vi "AxesControl.vi"(0 "Axis Up Down":string, 1 "Axis Left Right":string, 2 "Step size":dbl, 3 "Axis Up Down 2":string, 4 "Step size 2":dbl) -> ()   [LabVIEW 2014]
doc: "This VI allows the user to perform relative motion with a user defined step size of all every connected axis.\nThe VI sends messages in the name \"PI_Main\" queue that is also used by the FastAlignment_GUI as the main application.\nThis VI was designed for reentrant execution to allow the user to control more than three axes at once."
uses:
  C:/ProgramData/PI/LabVIEW/Low Level/General command.llb/Controller names.ctl
  Message Cluster.ctl
  C:/ProgramData/PI/LabVIEW/Low Level/General command.llb/Global2 (Array).vi
panel:
  out "Controller name":T1
  in  "stop":bool
  in  "System no.":i32=1 min=1 step=1
  in  "Up Down 2 Axis":u16(ring) items=["1", "2", "3", "4", "5", "6", "7", "8", "9", "10", "11", "12"]
  in  "Up Down Axis":u16(ring) items=["1", "2", "3", "4", "5", "6", "7", "8", "9", "10", "11", "12"]
  in  "Left Right Axis":u16(ring) items=["1", "2", "3", "4", "5", "6", "7", "8", "9", "10", "11", "12"]
  in  "Down Button 2":bool
  in  "Up Button 2":bool
  in  "Up Button":bool
  in  "Right Button":bool
  in  "Left Button":bool
  in  "Down Button":bool
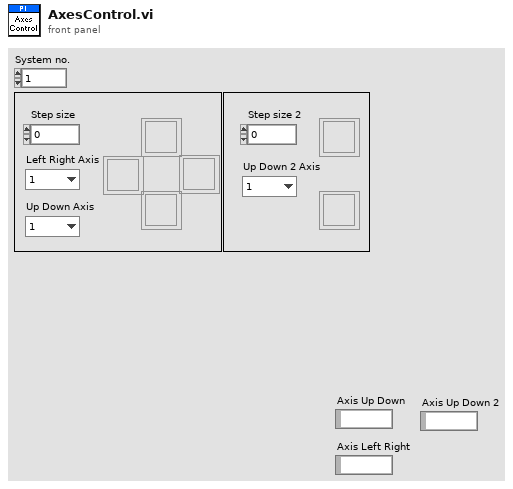
[diagram p1: front panel]
types:
  T1 = typedef "Controller names.ctl" = enum16{"None", "Analog", "C-702", "C-413", "C-414", "C-843", "C-843.PM", "C-844", "C-848", "C-865", "C-866", "C-867", "C-877", "C-880", "C-884", "C-885", "C-886", "C-887", "C-891", "E-135", "E-516", "E-517", "E-518", "E-709", "E-710", "E-712", "E-725", "E-727", "E-753", "E-754", "E-755", "E-761", "E-816", "E-861", "E-870", "E-871", "E-872", "E-873", "E-874", "F-206", "HydraPollux", "M-840", "M-850", "M-8X0", "Mercury", "Mercury_GCS", "PI_GCS2"}
  T2 = typedef "Message Cluster.ctl" = cluster{"Message":string, "Message Data":variant}
  T3 = cluster{"Conn. axes":string[], "Controller name":T1}[]
  T4 = cluster{"Conn. axes":string[], "Controller name":T1}
  T5 = cluster{"Axis":string, "Target":dbl, "System no.":i32}
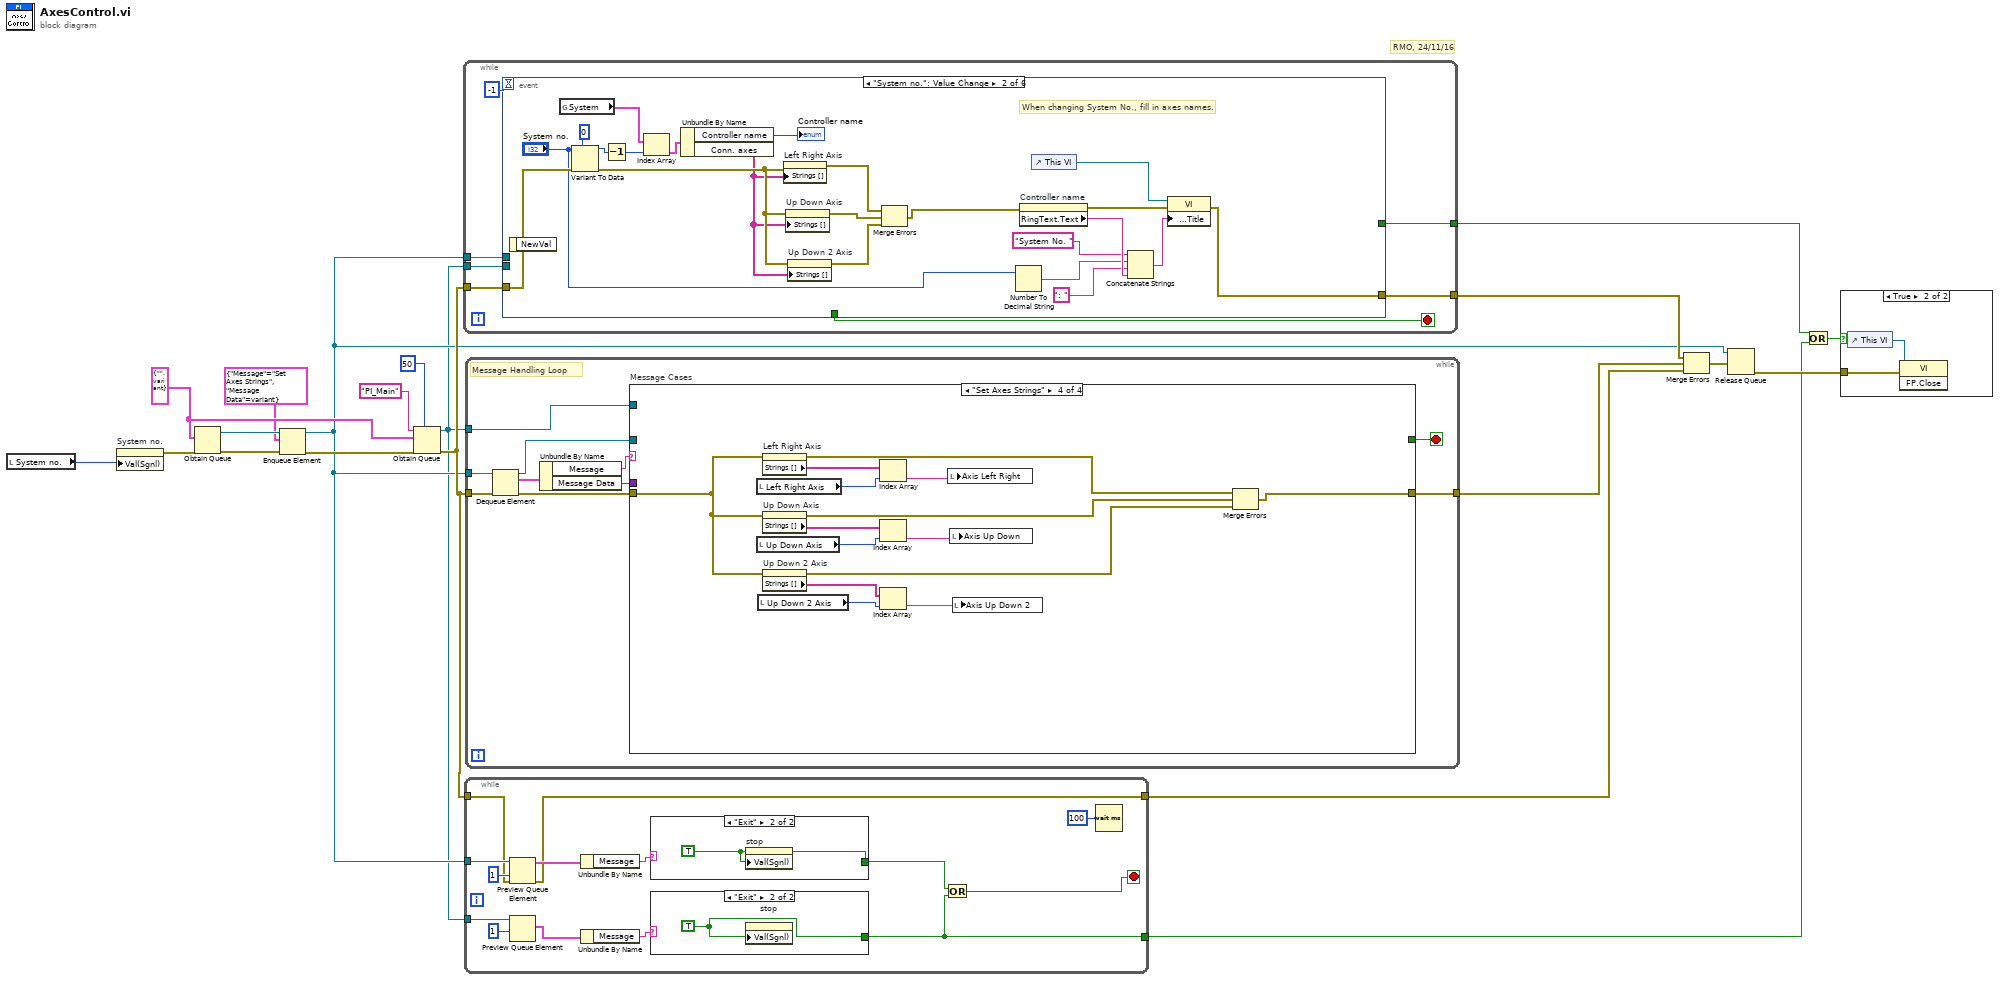
[diagram p0: block diagram]
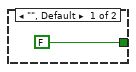
[diagram p3: hidden frame]
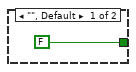
[diagram p4: hidden frame]
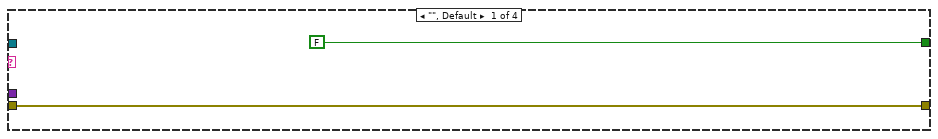
[diagram p5: hidden frame]
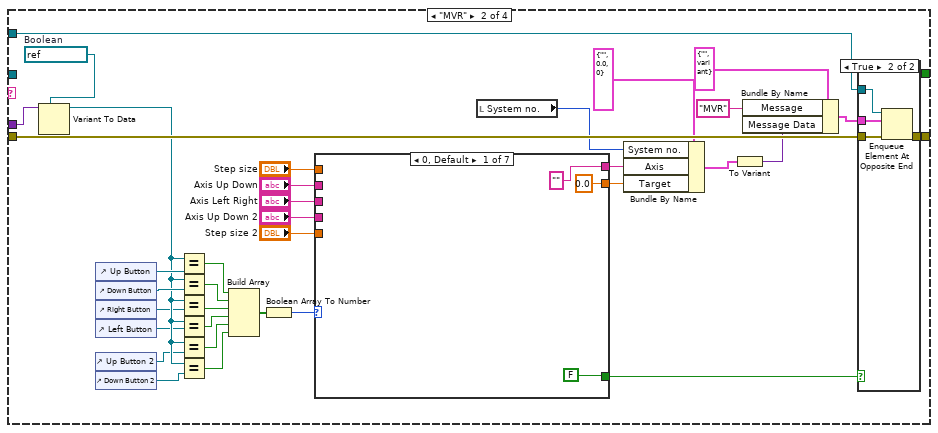
[diagram p6: hidden frame]
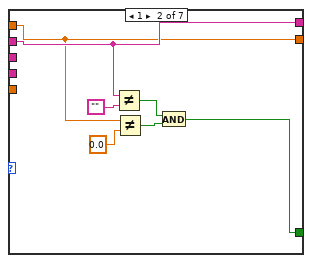
[diagram p8: hidden frame]
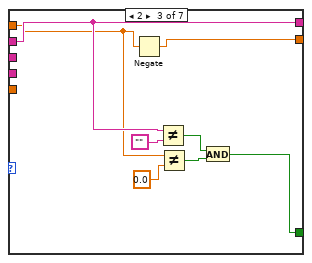
[diagram p9: hidden frame]
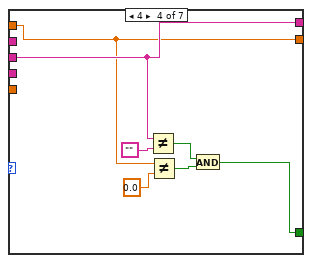
[diagram p10: hidden frame]
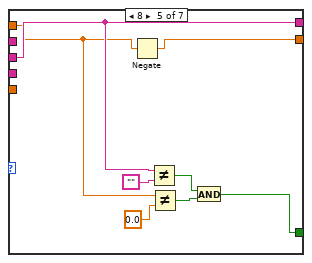
[diagram p11: hidden frame]
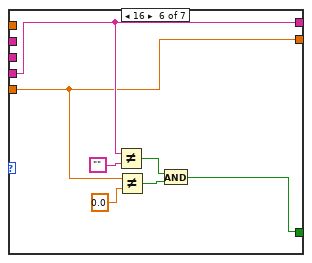
[diagram p12: hidden frame]
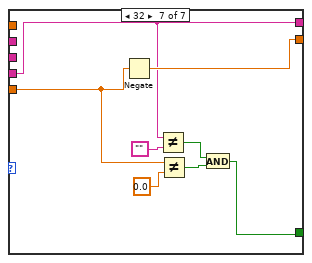
[diagram p13: hidden frame]
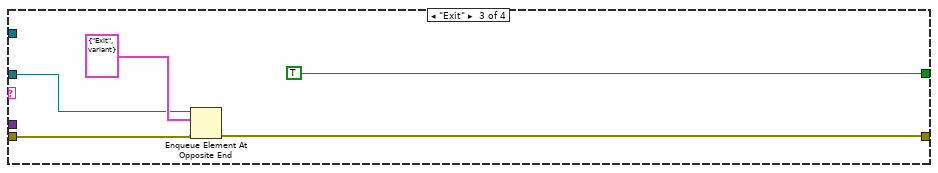
[diagram p14: hidden frame]
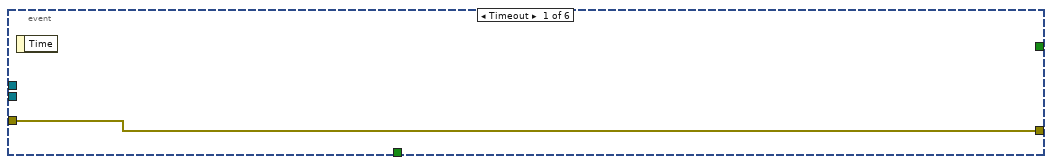
[diagram p15: hidden frame]
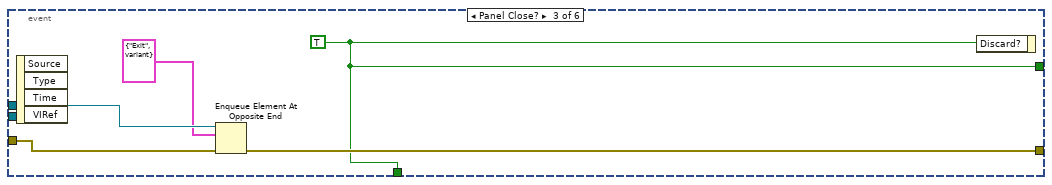
[diagram p16: hidden frame]
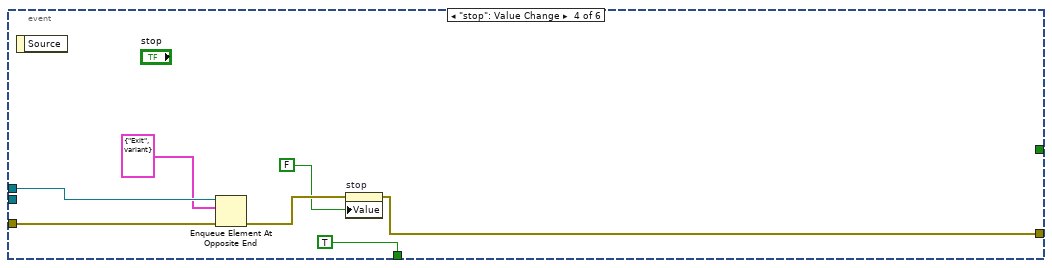
[diagram p17: hidden frame]
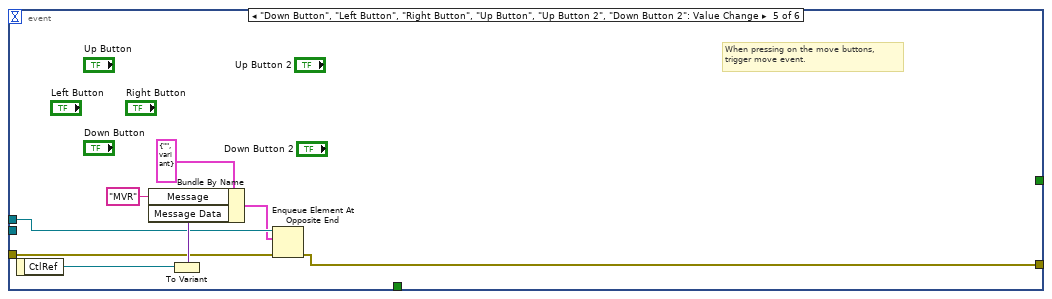
[diagram p18: hidden frame]
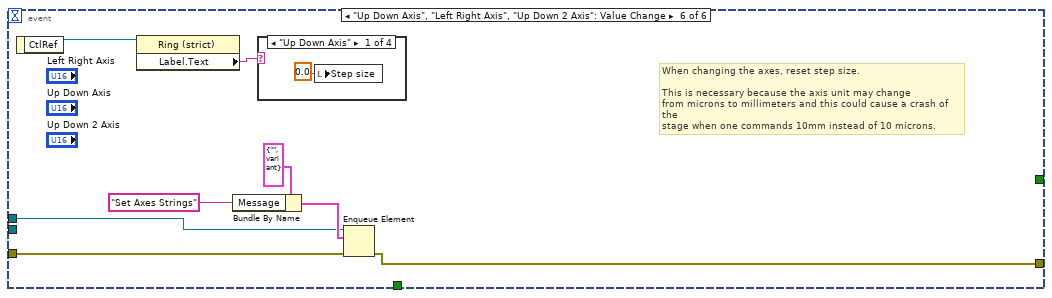
[diagram p19: hidden frame]
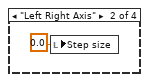
[diagram p20: hidden frame]
diagram:
  w18 = T2 {"Message"="", "Message Data"=variant} ("Message Cluster")
  # "RMO, 24/11/16"
  n1 = local read "System no."() -> (w1:i32)
  n2 = property on="System no." class="DigNum (strict)"("Val(Sgnl)"=w1) -> (error out=w2:errorcluster)  [unwired: 2 in, 1 out]
  n3 = Obtain Queue(element data type=w18, error in (no error)=w2) -> (queue out=w14:refnum<queue>, error out=w15:errorcluster)  [unwired: 2 in, 2 out]
  n4 = Enqueue Element(queue=w14, element=T2 {"Message"="Set Axes Strings", "Message Data"=variant} ("Message Cluster"), error in (no error)=w15) -> (queue out=w7:refnum<queue>, error out=w13:errorcluster)  [unwired: 2 out]
  n5 = Obtain Queue(max queue size (-1, unlimited)=50, name (unnamed)="PI_Main", element data type=w18, error in (no error)=w13) -> (queue out=w6:refnum<queue>, error out=w9:errorcluster)  [unwired: 1 in, 1 out]
  n6 = while {
    tunnel: [w27] -> w19
    tunnel: w6 -> [w26]
    tunnel: w9 -> [w24]
    tunnel: w7 -> [w22]
    tunnel: [w21] -> w5
    stop <- w25 stop-if-true
    n7 = event shown="[1] \"System no.\": Value Change" {
      selector: _ -> [_ _ _ _ _ _]
      dyn-events: _ -> [_ _ _ _ _ _]
      timeout: -1 -> [_ _ _ _ _ _]
      tunnel: [w28 w31 w53 w57 w70 w76] -> w27
      tunnel: w26 -> [_ _ _ _ _ _]
      tunnel: [_ _ w51 TRUE _ _] -> w25
      tunnel: w24 -> [w28 w40 w54 w61 w63 w74]
      tunnel: w22 -> [_ _ w55 w62 w66 w75]
      tunnel: [_ _ w51 _ _ _] -> w21
      event Timeout {
        n8 = event-data() -> ()  [unwired: 2 out]
      }
      event "System no.": Value Change {
        # "When changing System No., fill in axes names."
        n9 = event-data() -> ()  [unwired: 2 out]
        n10 = global read "Global2 (Array).vi" "System"() -> (w42:T3)
        n11 = Variant To Data(error in=w40, type=0, Variant="System no.") -> (data=w44:i32, error out=w47:errorcluster)
        n12 = Decrement(x=w44) -> (x-1=w45:i32)
        n13 = Index Array(array=w42, index=w45) -> (element=w43:T4)
        n14 = Unbundle By Name(w43) -> ("Controller name"=→"Controller name":T1, "Conn. axes"=w46:string[])
        n15 = property on="Left Right Axis" class="Ring (strict)"(error in=w47, "Strings []"=w46) -> (error out=w48:errorcluster)  [unwired: 1 in, 1 out]
        n16 = property on="Up Down Axis" class="Ring (strict)"(error in=w47, "Strings []"=w46) -> (error out=w49:errorcluster)  [unwired: 1 in, 1 out]
        n17 = property on="Up Down 2 Axis" class="Ring (strict)"(error in=w47, "Strings []"=w46) -> (error out=w50:errorcluster)  [unwired: 1 in, 1 out]
        n18 = Merge Errors(w48, w49, w50) -> (w32:errorcluster)
        n19 = Number To Decimal String(number="System no.") -> (decimal integer string=w36:string)  [unwired: 1 out]
        n20 = property on="Controller name" class="Enum (strict)"(error in=w32) -> (error out=w34:errorcluster, "RingText.Text"=w39:string)  [unwired: 1 in, 1 out]
        n21 = control-ref of="This VI"() -> (w33:refnum<vi>)
        n22 = Concatenate Strings("System No. ", w36, ": " ("string"), w39) -> (w38:string)
        n23 = property class="VI"(reference=w33, error in=w34, "Front Panel.Title"=w38) -> (error out=w31:errorcluster)  [unwired: 1 out]
      }
      event Panel Close? {
        w51 = TRUE
        n24 = event-data() -> ()  [unwired: 5 out]
        n25 = Enqueue Element At Opposite End(queue=w55, element=T2 {"Message"="Exit", "Message Data"=variant}, error in (no error)=w54) -> (error out=w53:errorcluster)  [unwired: 3 out]
        n26 = event-data("Discard?"=w51) -> ()  [unwired: 1 in, 1 out]
      }
      event "stop": Value Change {
        n27 = event-data() -> ()  [unwired: 2 out]
        n28 = Enqueue Element At Opposite End(queue=w62, element=T2 {"Message"="Exit", "Message Data"=variant}, error in (no error)=w61) -> (error out=w59:errorcluster)  [unwired: 3 out]
        n29 = property on="stop" class="Bool (strict)"(error in=w59, "Value"=FALSE) -> (error out=w57:errorcluster)  [unwired: 1 in, 1 out]
      }
      event "Down Button", "Left Button", "Right Button", "Up Button", "Up Button 2", "Down Button 2": Value Change {
        # "When pressing on the move buttons,\ntrigger move event."
        n30 = event-data() -> ("CtlRef"=w64:refnum<vi>)  [unwired: 1 out]
        n31 = To Variant(anything=w64) -> (Variant=w68:variant)
        n32 = Bundle By Name(cluster=T2 {"Message"="", "Message Data"=variant} ("Message Cluster"), "Message"="MVR", "Message Data"=w68) -> (w65:T2)
        n33 = Enqueue Element At Opposite End(queue=w66, element=w65, error in (no error)=w63) -> (error out=w70:errorcluster)  [unwired: 3 out]
      }
      event "Up Down Axis", "Left Right Axis", "Up Down 2 Axis": Value Change {
        # "When changing the axes, reset step size.\n\nThis is necessary because the axis unit may change\nfrom microns to millimeters and this could cause a crash of the\nstage when one commands 10mm instead of 10 microns."
        n34 = event-data() -> ("CtlRef"=w72:refnum<vi>)  [unwired: 1 out]
        n35 = property class="Ring (strict)"(reference=w72) -> ("Label.Text"=w71:string)  [unwired: 1 in, 2 out]
        n36 = Bundle By Name(cluster=T2 {"Message"="", "Message Data"=variant} ("Message Cluster"), "Message"="Set Axes Strings") -> (w77:T2)
        n37 = case shown="\"Up Down Axis\"" w71 {
          frame "Up Down Axis" {
            n38 = local write "Step size"(0.0 ("Step size")) -> ()
          }
          frame "Left Right Axis" {
            n39 = local write "Step size"(0.0 ("Step size")) -> ()
          }
          frame "", Default {
          }
          frame "Up Down 2 Axis" {
            n40 = local write "Step size 2"(0.0 ("Step size")) -> ()
          }
        }
        n41 = Enqueue Element(queue=w75, element=w77, error in (no error)=w74) -> (error out=w76:errorcluster)  [unwired: 3 out]
      }
    }
  }
  n42 = while {
    tunnel: w7 -> [w92]
    tunnel: w9 -> [w90]
    tunnel: [w89] -> w8
    tunnel: w6 -> [w85]
    tunnel: [w82] -> w4
    stop <- w86 stop-if-true
    n43 = Preview Queue Element(queue=w92, timeout in ms (-1)=1, error in (no error)=w90) -> (element=w95:T2, error out=w89:errorcluster)  [unwired: 2 out]
    n44 = Preview Queue Element(queue=w85, timeout in ms (-1)=1) -> (element=w84:T2)  [unwired: 1 in, 3 out]
    n45 = Unbundle By Name(w95) -> ("Message"=w94:string)
    n46 = Unbundle By Name(w84) -> ("Message"=w88:string)
    n47 = case shown="\"Exit\"" w94 {
      tunnel: [FALSE w99] -> w87
      frame "", Default {
      }
      frame "Exit" {
        w99 = TRUE
        n48 = property on="stop" class="Bool (strict)"("Val(Sgnl)"=w99) -> ()  [unwired: 2 in, 2 out]
      }
    }
    n49 = case shown="\"Exit\"" w88 {
      tunnel: [FALSE w97] -> w82
      frame "", Default {
      }
      frame "Exit" {
        w97 = TRUE
        n50 = property on="stop" class="Bool (strict)"("Val(Sgnl)"=w97) -> ()  [unwired: 2 in, 2 out]
      }
    }
    n51 = Or(x=w87, y=w82) -> (x .or. y?=w86:bool)
    n52 = Wait (ms)(milliseconds to wait=u32 100) -> ()  [unwired: 1 out]
  }
  n53 = while {
    tunnel: w7 -> [w101]
    tunnel: w9 -> [w107]
    tunnel: [w108] -> w17
    tunnel: w6 -> [w102]
    stop <- w109 stop-if-true
    # "Message Handling Loop"
    n54 = Dequeue Element(queue=w101, error in (no error)=w107) -> (queue out=w100:refnum<queue>, element=w106:T2, error out=w105:errorcluster)  [unwired: 2 out]
    n55 = Unbundle By Name(w106) -> ("Message"=w104:string, "Message Data"=w103:variant)
    n56 = case "Message Cases" shown="\"Set Axes Strings\"" w104 {
      tunnel: w105 -> [w111 w146 w203 w212]
      tunnel: [w111 w145 w202 w205] -> w108
      tunnel: [FALSE _ TRUE _] -> w109
      tunnel: w103 -> [_ w135 _ _]
      tunnel: w102 -> [_ w144 _ _]
      tunnel: w100 -> [_ _ w200 _]
      frame "", Default {
      }
      frame "MVR" {
        w137 = refnum<vi> refnum  # Boolean
        n57 = Variant To Data(type=w137, Variant=w135) -> (data=w133:refnum<vi>)  [unwired: 1 in, 1 out]
        n58 = control-ref of="Up Button"() -> (w136:refnum<vi>)
        n59 = control-ref of="Down Button"() -> (w134:refnum<vi>)
        n60 = control-ref of="Right Button"() -> (w114:refnum<vi>)
        n61 = control-ref of="Left Button"() -> (w113:refnum<vi>)
        n62 = control-ref of="Up Button 2"() -> (w118:refnum<vi>)
        n63 = control-ref of="Down Button 2"() -> (w117:refnum<vi>)
        n64 = Equal?(x=w133, y=w136) -> (x = y?=w132:bool)
        n65 = Equal?(x=w133, y=w134) -> (x = y?=w131:bool)
        n66 = Equal?(x=w133, y=w114) -> (x = y?=w130:bool)
        n67 = Equal?(x=w133, y=w113) -> (x = y?=w129:bool)
        n68 = Equal?(x=w133, y=w118) -> (x = y?=w128:bool)
        n69 = Equal?(x=w133, y=w117) -> (x = y?=w127:bool)
        n70 = Build Array(w132, w131, w130, w129, w128, w127) -> (w126:bool[])
        n71 = Boolean Array To Number(Boolean array=w126) -> (number=w122:u32)
        n72 = case shown="0, Default" w122 {
          tunnel: "Step size" -> [_ w156 w163 w171 w178 _ _]
          tunnel: "Axis Up Down" -> [_ w157 w164 _ _ _ _]
          tunnel: "Axis Left Right" -> [_ _ _ w172 w179 _ _]
          tunnel: "Axis Up Down 2" -> [_ _ _ _ _ w187 w194]
          tunnel: "Step size 2" -> [_ _ _ _ _ w186 w193]
          tunnel: [FALSE w155 w162 w170 w177 w185 w192] -> w121
          tunnel: ["" w157 w164 w172 w179 w187 w194] -> w116
          tunnel: [0.0 ("Step size 2") w156 w169 w171 w184 w186 w199] -> w115
          frame 0, Default {
          }
          frame 1 {
            n73 = Not Equal?(x=w157, y="") -> (x != y?=w159:bool)
            n74 = Not Equal?(x=w156, y=0.0 ("Step size")) -> (x != y?=w158:bool)
            n75 = And(x=w159, y=w158) -> (x .and. y?=w155:bool)
          }
          frame 2 {
            n76 = Negate(x=w163) -> (-x=w169:dbl)
            n77 = Not Equal?(x=w164, y="") -> (x != y?=w166:bool)
            n78 = Not Equal?(x=w163, y=0.0 ("Step size")) -> (x != y?=w165:bool)
            n79 = And(x=w166, y=w165) -> (x .and. y?=w162:bool)
          }
          frame 4 {
            n80 = Not Equal?(x=w172, y="") -> (x != y?=w174:bool)
            n81 = Not Equal?(x=w171, y=0.0 ("Step size")) -> (x != y?=w173:bool)
            n82 = And(x=w174, y=w173) -> (x .and. y?=w170:bool)
          }
          frame 8 {
            n83 = Negate(x=w178) -> (-x=w184:dbl)
            n84 = Not Equal?(x=w179, y="") -> (x != y?=w181:bool)
            n85 = Not Equal?(x=w178, y=0.0 ("Step size")) -> (x != y?=w180:bool)
            n86 = And(x=w181, y=w180) -> (x .and. y?=w177:bool)
          }
          frame 16 {
            n87 = Not Equal?(x=w187, y="") -> (x != y?=w189:bool)
            n88 = Not Equal?(x=w186, y=0.0 ("Step size")) -> (x != y?=w188:bool)
            n89 = And(x=w189, y=w188) -> (x .and. y?=w185:bool)
          }
          frame 32 {
            n90 = Negate(x=w193) -> (-x=w199:dbl)
            n91 = Not Equal?(x=w194, y="") -> (x != y?=w196:bool)
            n92 = Not Equal?(x=w193, y=0.0 ("Step size")) -> (x != y?=w195:bool)
            n93 = And(x=w196, y=w195) -> (x .and. y?=w192:bool)
          }
        }
        n94 = local read "System no."() -> (w112:i32)
        n95 = Bundle By Name(cluster=T5 {"Axis"="", "Target"=0.0, "System no."=0}, "System no."=w112, "Axis"=w116, "Target"=w115) -> (w142:T5)
        n96 = To Variant(anything=w142) -> (Variant=w140:variant)
        n97 = Bundle By Name(cluster=T2 {"Message"="", "Message Data"=variant} ("Message Cluster"), "Message"="MVR", "Message Data"=w140) -> (w138:T2)
        n98 = case shown="True" w121 {
          tunnel: w146 -> [w147 w151]
          tunnel: [w147 w150] -> w145
          tunnel: w144 -> [_ w149]
          tunnel: w138 -> [_ w148]
          frame False {
          }
          frame True {
            n99 = Enqueue Element At Opposite End(queue=w149, element=w148, error in (no error)=w151) -> (error out=w150:errorcluster)  [unwired: 3 out]
          }
        }
      }
      frame "Exit" {
        n100 = Enqueue Element At Opposite End(queue=w200, element=T2 {"Message"="Exit", "Message Data"=variant}, error in (no error)=w203) -> (error out=w202:errorcluster)  [unwired: 3 out]
      }
      frame "Set Axes Strings" {
        n101 = local read "Left Right Axis"() -> (w217:u16)
        n102 = local read "Up Down Axis"() -> (w215:u16)
        n103 = local read "Up Down 2 Axis"() -> (w213:u16)
        n104 = property on="Left Right Axis" class="Ring (strict)"(error in=w212) -> (error out=w208:errorcluster, "Strings []"=w218:string[])  [unwired: 1 in, 1 out]
        n105 = property on="Up Down Axis" class="Ring (strict)"(error in=w212) -> (error out=w207:errorcluster, "Strings []"=w216:string[])  [unwired: 1 in, 1 out]
        n106 = property on="Up Down 2 Axis" class="Ring (strict)"(error in=w212) -> (error out=w206:errorcluster, "Strings []"=w214:string[])  [unwired: 1 in, 1 out]
        n107 = Index Array(array=w218, index=w217) -> (element=w211:string)
        n108 = Index Array(array=w216, index=w215) -> (element=w210:string)
        n109 = Index Array(array=w214, index=w213) -> (element=w209:string)
        n110 = local write "Axis Left Right"(w211) -> ()
        n111 = local write "Axis Up Down"(w210) -> ()
        n112 = local write "Axis Up Down 2"(w209) -> ()
        n113 = Merge Errors(w208, w207, w206) -> (w205:errorcluster)
      }
    }
  }
  n114 = Merge Errors(w19, w17, w8) -> (w16:errorcluster)
  n115 = Release Queue(queue=w7, error in (no error)=w16) -> (error out=w10:errorcluster)  [unwired: 3 out]
  n116 = Or(x=w5, y=w4) -> (x .or. y?=w3:bool)
  n117 = case shown="True" w3 {
    tunnel: w10 -> [_ w219]
    frame False {
    }
    frame True {
      n118 = control-ref of="This VI"() -> (w220:refnum<vi>)
      n119 = invoke class="VI" method="FP.Close"(reference=w220, error in=w219) -> ()  [unwired: 1 in, 3 out]
    }
  }
